vi "Convert data stream.vi"(1 "n floats":i32=10 min=0 max=256, 2 "Floats only (starting byte index 3)":string) -> (0 "Data":sgl[](array[numeric]))   [LabVIEW 2017]
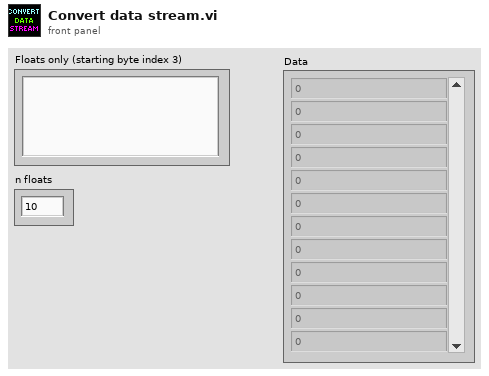
[diagram p1: front panel]
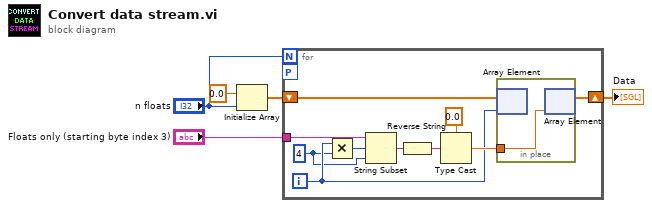
[diagram p0: block diagram]
diagram:
  n1 = Initialize Array(sgl 0.0, "n floats") -> (w4:sgl[])
  n2 = for {
    N: "n floats" -> [_]
    tunnel: "Floats only (starting byte index 3)" -> [w12]
    shift-right: [w8] -> w1
    shift-left: w4 -> [w10]
    workers-P: _ -> [_]
    i -> [w7]
    w6 = 4 ("x")
    n3 = Multiply(x=w7, y=w6) -> (x*y=w11:i32)
    n4 = String Subset(string=w12, offset (0)=w11, length (rest)=w6) -> (substring=w13:string)
    n5 = Reverse String(1:w13) -> (0:w14:string)
    n6 = Type Cast(type=sgl 0.0, x=w14) -> (*(type *) &x=w9:sgl)
    n7 = in-place {
      in-place-border: w9 -> [w16]
      n8 = in-place-array #1(w10, w7) -> ()  [unwired: 1 out]
      n9 = in-place-array #1(w16) -> (w8:sgl[])  [unwired: 1 out]
    }
  }
  "Data" <- w1
